vi "Event Handler.vi"(8 "error in (no error)":errorcluster, 10 "Stop Event Handler":refnum<user-event>, 11 "QControl_Graph in":refnum<class "QControl_Graph.lvclass">) -> (0 "error out":errorcluster)   [LabVIEW 2017, in "QControl_Graph.lvclass"]
doc: "The <b>Event Handler VI</b> is a dynamic dispatch VI that should be overwritten if events are needed to create the enhanced QControl. \n\nBy inheriting from the main Control.lvclass the overwritten <b>Event Handler VI</b> will be launched asynchronously in the initialization of the QControl.\n<b> </b> <b> </b>\n©2016 Q Software Innovations, LLC (QSI)\nwritten by Quentin Alldredge\nproduced in LabVIEW 2015\n\nsupport@qsoftwareinnovations.com\nwww.qsoftwareinnovations.com\n\nAll rights reserved.\n\nRedistribution and use in source and binary forms, with or without modification, are permitted provided that the following conditions are met:\n\n * Redistributions of source code must retain the above copyright notice, this list of conditions and the following disclaimer.\n * Redistributions in binary form must reproduce the above copyright notice, this list of conditions and the following disclaimer in the documentation and/or other materials provided with the distribution.\n * Neither the name of Q Software Innovations, LLC. nor the names of its contributors may be used to endorse or promote products derived from this software without specific prior written permission.\n\nTHIS SOFTWARE IS PROVIDED BY THE COPYRIGHT HOLDERS AND CONTRIBUTORS \"AS IS\" AND ANY EXPRESS OR IMPLIED WARRANTIES, INCLUDING, BUT NOT LIMITED TO, THE IMPLIED WARRANTIES OF MERCHANTABILITY AND FITNESS FOR A PARTICULAR PURPOSE ARE DISCLAIMED. IN NO EVENT SHALL THE COPYRIGHT OWNER OR CONTRIBUTORS BE LIABLE FOR ANY DIRECT, INDIRECT, INCIDENTAL, SPECIAL, EXEMPLARY, OR CONSEQUENTIAL DAMAGES (INCLUDING, BUT NOT LIMITED TO, PROCUREMENT OF SUBSTITUTE GOODS OR SERVICES; LOSS OF USE, DATA, OR PROFITS; OR BUSINESS INTERRUPTION) HOWEVER CAUSED AND ON ANY THEORY OF LIABILITY, WHETHER IN CONTRACT, STRICT LIABILITY, OR TORT (INCLUDING NEGLIGENCE OR OTHERWISE) ARISING IN ANY WAY OUT OF THE USE OF THIS SOFTWARE, EVEN IF ADVISED OF THE POSSIBILITY OF SUCH DAMAGE."
uses:
  QControl_Graph.lvclass
  C:/Program Files (x86)/National Instruments/LabVIEW 2017/vi.lib/QSI/QControls/QControl Classes/WaveformGraph/WaveformGraph.lvclass
  QControl_Graph.lvclass/QControl_Graph.ctl
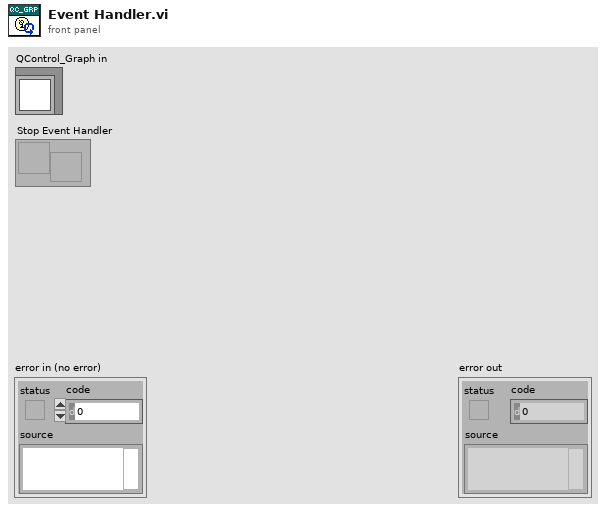
[diagram p1: front panel]
types:
  T1 = cluster{"Shift":bool, "Ctrl":bool, "Alt":bool, "Cmd":bool, "Opt":bool}
  T2 = typedef "LVPoint32TypeDef.ctl" = cluster{"Horizontal":i32, "Vertical":i32}
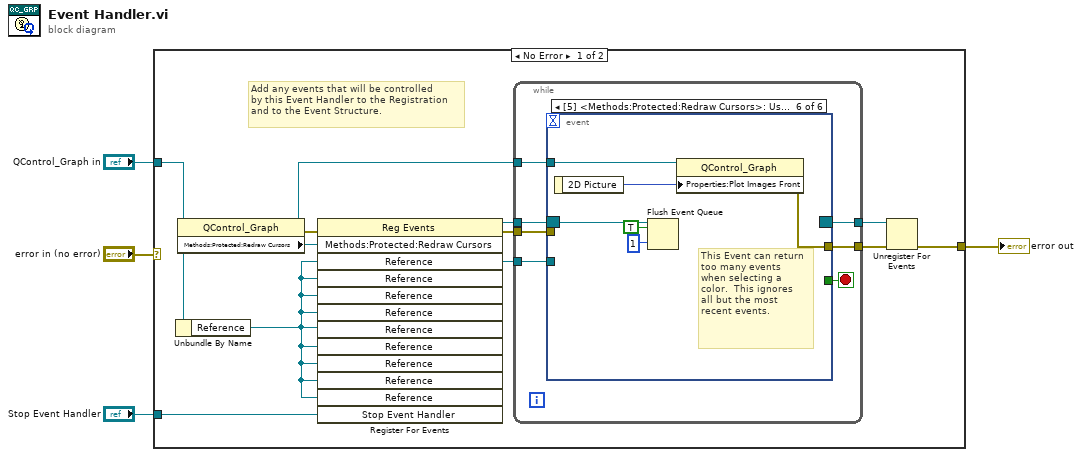
[diagram p0: block diagram]
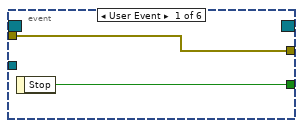
[diagram p2: hidden frame]
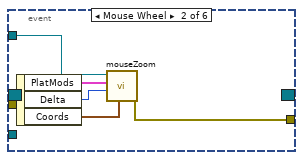
[diagram p3: hidden frame]
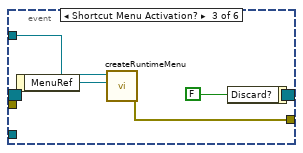
[diagram p4: hidden frame]
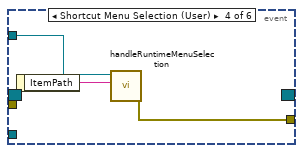
[diagram p5: hidden frame]
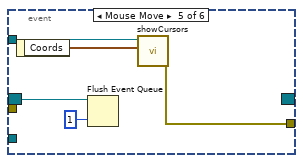
[diagram p6: hidden frame]
diagram:
  n1 = case shown="No Error" "error in (no error)" {
    selector: "error in (no error)" -> [_ w48]
    tunnel: [w12 w48] -> w3
    tunnel: "QControl_Graph in" -> [w8 _]
    tunnel: "Stop Event Handler" -> [w10 _]
    frame No Error {
      # "Add any events that will be controlled\nby this Event Handler to the Registration\nand to the Event Structure."
      n2 = Unbundle By Name(w8) -> ("Reference"=w9:refnum<vi>)
      n3 = property class="QControl_Graph"(reference=w8) -> (reference out=w7:refnum<class "QControl_Graph.lvclass">, error out=w5:errorcluster, "Methods:Protected:Redraw Cursors"=w6:refnum<user-event>)  [unwired: 1 in]
      n4 = register-events(error in=w5, w6, w9, w9, w9, w9, w9, w9, w9, w9, w9, w10) -> (reference out=w15:refnum<event-registration>, error out=w14:errorcluster)  [unwired: 1 in]
      n5 = while {
        tunnel: w15 -> [w22]
        tunnel: w14 -> [w20]
        tunnel: [w19] -> w13
        tunnel: [w17] -> w11
        tunnel: w9 -> [w16]
        tunnel: w7 -> [w21]
        stop <- w18 stop-if-true
        n6 = event shown="[5] <Methods:Protected:Redraw Cursors>: User Event" {
          selector: w22 -> [_ _ _ _ w37 w43]
          dyn-events: [_ _ _ _ _ _] -> w17
          timeout: _ -> [_ _ _ _ _ _]
          tunnel: w21 -> [_ w29 w32 w36 w41 w47]
          tunnel: w20 -> [w24 _ _ _ _ _]
          tunnel: [w24 w25 w31 w35 w40 w45] -> w19
          tunnel: [w23 _ _ _ _ _] -> w18
          tunnel: w16 -> [_ _ _ _ _ _]
          event User Event {
            n7 = event-data() -> ("Stop"=w23:bool)  [unwired: 1 in]
          }
          event Mouse Wheel {
            n8 = event-data() -> ("PlatMods"=w28:T1, "Delta"=w27:i32, "Coords"=w26:T2)  [unwired: 1 in]
            n9 = call-dynamic "mouseZoom.vi"("XY"=w26, "Delta"=w27, "PlatMods"=w28, "QControl_Graph in"=w29) -> ("error out"=w25:errorcluster)  [unwired: 6 in, 1 out]
          }
          event Shortcut Menu Activation? {
            n10 = event-data() -> ("MenuRef"=w33:refnum<k9>)  [unwired: 1 in]
            n11 = call "createRuntimeMenu.vi"("menu reference"=w33, "QControl_Graph in"=w32) -> ("error out"=w31:errorcluster)  [unwired: 8 in, 1 out]
            n12 = event-data("Discard?"=FALSE) -> ()  [unwired: 1 in, 1 out]
          }
          event Shortcut Menu Selection (User) {
            n13 = event-data() -> ("ItemPath"=w34:string)  [unwired: 1 in]
            n14 = call "handleRuntimeMenuSelection.vi"("ItemPath"=w34, "QControl_Graph in"=w36) -> ("error out"=w35:errorcluster)  [unwired: 8 in, 1 out]
          }
          event Mouse Move {
            n15 = event-data() -> ("Coords"=w39:T2)  [unwired: 1 in]
            n16 = Flush Event Queue(0:w37, 5:1 ("keep most recent")) -> ()  [unwired: 4 in, 3 out]
            n17 = call-dynamic "showCursors.vi"("XY"=w39, "QControl_Graph in"=w41) -> ("error out"=w40:errorcluster)  [unwired: 8 in, 1 out]
          }
          event User Event {
            # "This Event can return\ntoo many events\nwhen selecting a \ncolor.  This ignores \nall but the most\nrecent events."
            n18 = event-data() -> ("2D Picture"=w46:picture)  [unwired: 1 in]
            n19 = Flush Event Queue(0:w43, 1:TRUE ("include static events? (T)"), 5:1 ("keep most recent")) -> ()  [unwired: 3 in, 3 out]
            n20 = property class="QControl_Graph"(reference=w47, "Properties:Plot Images Front"=w46) -> (error out=w45:errorcluster)  [unwired: 1 in, 1 out]
          }
        }
      }
      n21 = Unregister For Events(event registration refnum=w11, error in=w13) -> (error out=w12:errorcluster)
    }
    frame Error {
    }
  }
  "error out" <- w3
